vi "SUB SingleTrialPLV_v03.vi"(9 "fc":dbl, 10 "Theta":cluster{"Lat":dbl, "Length":dbl}={"Lat"=5.0, "Length"=60.0}, 11 "Waveform":waveform(dbl)) -> (0 "Instantaneous Phase":waveform(dbl), 1 "phase":dbl[](array[numeric]), 2 "PLV graph":cluster{dbl[], dbl[]}[](graph), 3 "PLV":dbl, 4 "Vector":dbl[](array[numeric]))   [LabVIEW 2017]
panel:
  out "dt":dbl
  in  "N 2":i32
  out "BinSize":i32
  out "N":i32
  out "M":i32
  out "N":i32
  out "y":dbl
  out "x":dbl
  out "PLV graph 2":cluster{dbl[], dbl[]}(graph)
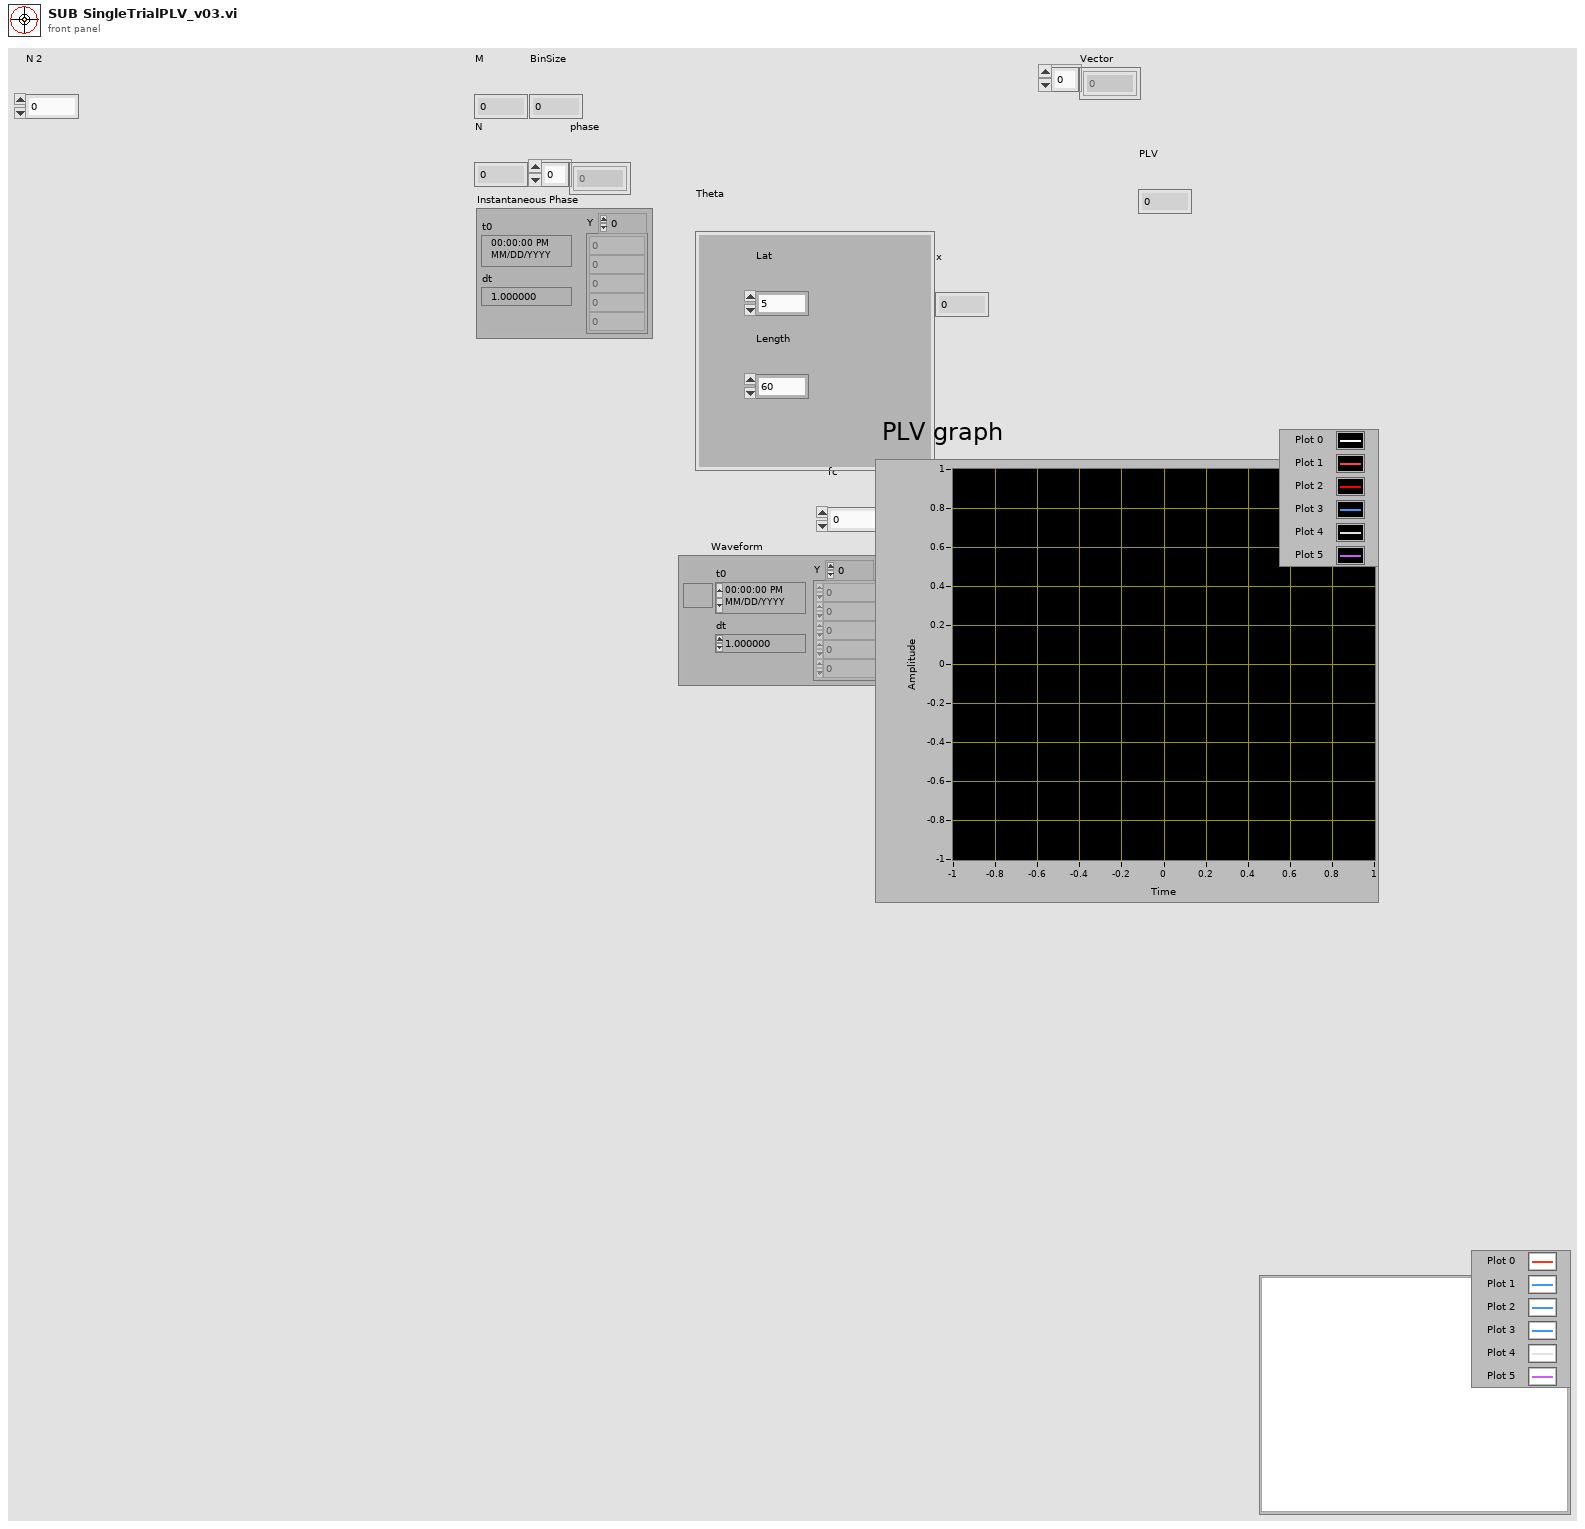
[diagram p1: front panel]
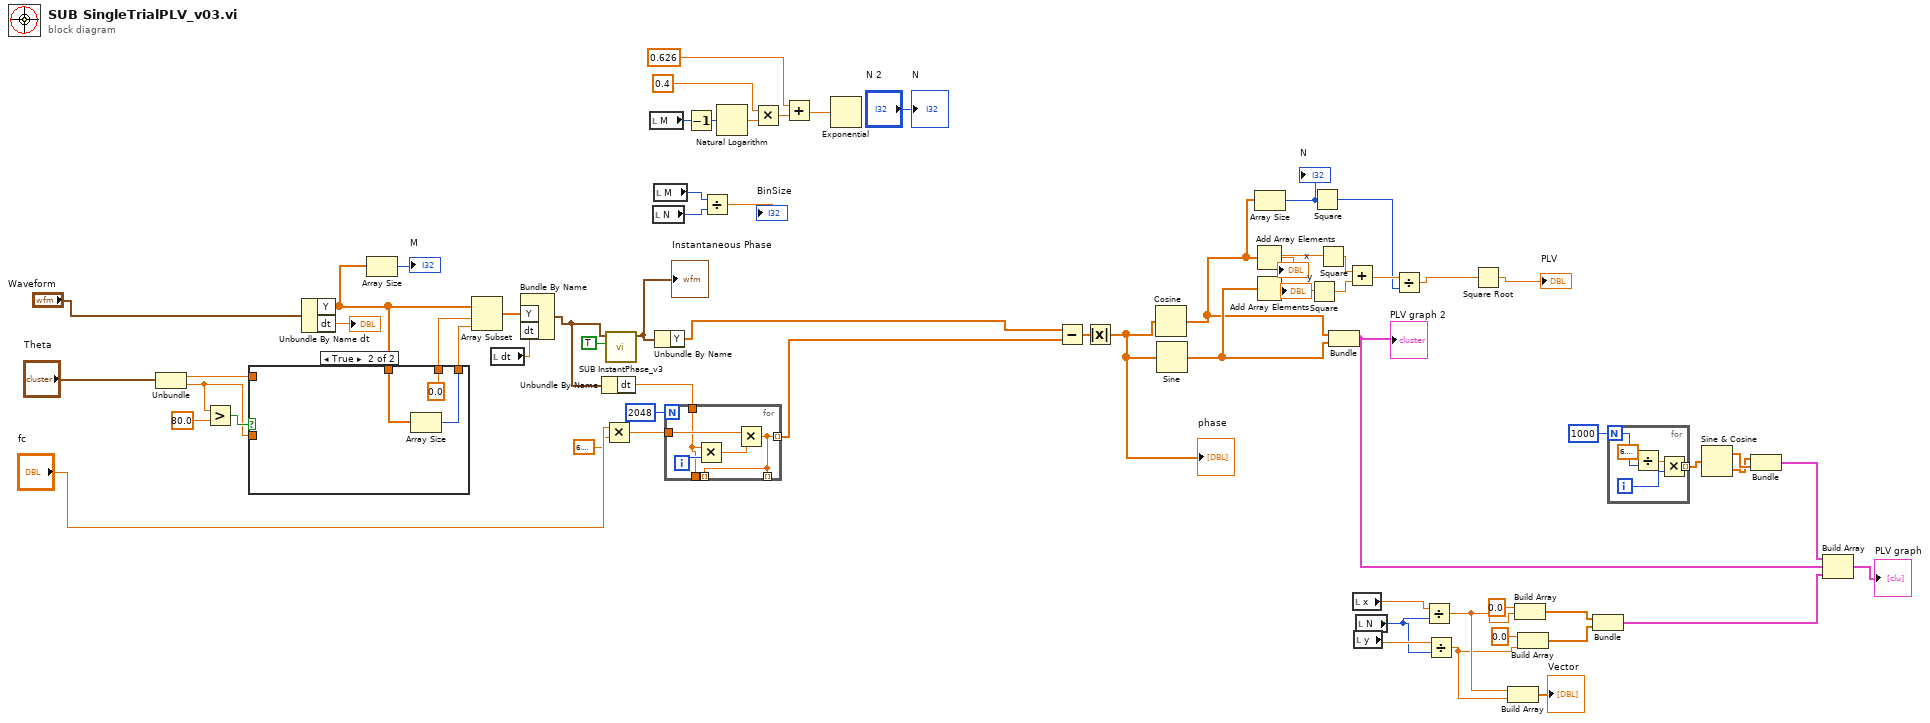
[diagram p0: block diagram]
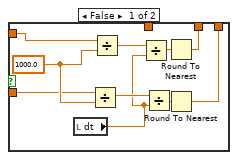
[diagram p2: hidden frame]
diagram:
  n1 = Unbundle("Theta") -> ("Lat"=w47:dbl, "Length"=w6:dbl)
  n2 = Greater?(x=w6, y=80.0) -> (0:w8:bool)
  n3 = Unbundle By Name("Waveform") -> ("Y"=w7:dbl[], "dt"=→"dt":dbl)
  n4 = case shown="True" w8 {
    tunnel: w47 -> [w75 _]
    tunnel: [w69 0.0] -> w46
    tunnel: [w68 w77] -> w43
    tunnel: w7 -> [_ w76]
    tunnel: w6 -> [w66 _]
    frame False {
      w74 = 1000.0 ("y")
      n5 = local read "dt"() -> (w67:dbl)
      n6 = Divide(x=w66, y=w74) -> (x/y=w72:dbl)
      n7 = Divide(x=w75, y=w74) -> (x/y=w73:dbl)
      n8 = Divide(x=w73, y=w67) -> (x/y=w71:dbl)
      n9 = Divide(x=w72, y=w67) -> (x/y=w70:dbl)
      n10 = Round To Nearest(number=w71) -> (nearest integer value=w69:dbl)
      n11 = Round To Nearest(number=w70) -> (nearest integer value=w68:dbl)
    }
    frame True {
      n12 = Array Size(array=w76) -> (size(s)=w77:i32)
    }
  }
  n13 = Array Size(array=w7) -> (size(s)=→"M":i32)
  n14 = Array Subset(array=w7, index=w46, length=w43) -> (w45:dbl[])
  n15 = local read "dt"() -> (w9:dbl)
  n16 = Bundle By Name("Y"=w45, "dt"=w9) -> (w44:waveform(dbl))  [unwired: 1 in]
  n17 = Unbundle By Name(w44) -> ("dt"=w60:dbl)
  n18 = Multiply(x="fc", y=6.283185307179586) -> (x*y=w62:dbl)
  n19 = call "SUB InstantPhase_v3.vi"("Unwrap"=TRUE, "Waveform"=w44) -> ("Instantaneous Phase"=w59:waveform(dbl))  [unwired: 9 in]
  "Instantaneous Phase" <- w59
  n20 = local read "M"() -> (w24:i32)
  n21 = local read "N"() -> (w16:i32)
  n22 = local read "M"() -> (w17:i32)
  n23 = Unbundle By Name(w59) -> ("Y"=w12:dbl[])
  n24 = for {
    N: 2048 -> [_]
    tunnel: w62 -> [w82]
    tunnel: w60 -> [w79]
    tunnel: [w80] -> w13 mode=indexing
    tunnel: [w80] -> _ mode=indexing
    tunnel: [w80] -> _ mode=indexing
    tunnel: [w79] -> _
    i -> [w83]
    n25 = Multiply(x=w79, y=w83) -> (x*y=w81:dbl)
    n26 = Multiply(x=w82, y=w81) -> (x*y=w80:dbl)
  }
  n27 = Decrement(x=w24) -> (x-1=w23:i32)
  n28 = Divide(x=w17, y=w16) -> (x/y=→"BinSize":dbl)
  n29 = Natural Logarithm(1:w23) -> (0:w22:dbl)
  n30 = Multiply(x=0.4, y=w22) -> (x*y=w20:dbl)
  n31 = Add(x=0.626, y=w20) -> (x+y=w18:dbl)
  n32 = Exponential(1:w18) -> ()  [unwired: 1 out]
  n33 = Subtract(x=w12, y=w13) -> (x-y=w58:dbl[])
  n34 = Absolute Value(x=w58) -> (abs(x)=w2:dbl[])
  "phase" <- w2
  n35 = Cosine(x=w2) -> (cos(x)=w51:dbl[])
  n36 = Sine(x=w2) -> (sin(x)=w57:dbl[])
  n37 = Add Array Elements(numeric array=w51) -> (sum=w56:dbl)
  "x" <- w56
  n38 = Add Array Elements(numeric array=w57) -> (sum=w55:dbl)
  "y" <- w55
  n39 = Array Size(array=w51) -> (size(s)=w49:i32)
  "N" <- w49
  n40 = Square(x=w55) -> (x^2=w53:dbl)
  n41 = Square(x=w49) -> (x^2=w48:i32)
  n42 = Square(x=w56) -> (x^2=w54:dbl)
  n43 = Bundle(w51, w57) -> (w35:cluster{dbl[], dbl[]})  [unwired: 1 in]
  "PLV graph 2" <- w35
  n44 = Add(x=w54, y=w53) -> (x+y=w52:dbl)
  n45 = local read "x"() -> (w34:dbl)
  n46 = local read "y"() -> (w28:dbl)
  n47 = local read "N"() -> (w27:i32)
  n48 = Divide(x=w52, y=w48) -> (x/y=w50:dbl)
  n49 = Divide(x=w34, y=w27) -> (x/y=w5:dbl)
  n50 = Divide(x=w28, y=w27) -> (x/y=w4:dbl)
  n51 = Square Root(x=w50) -> (sqrt(x)=→"PLV":dbl)
  n52 = Build Array(w5, w4) -> (→"Vector":dbl[])
  n53 = Build Array(0.0 ("element"), w5) -> (w31:dbl[])
  n54 = Build Array(0.0 ("element"), w4) -> (w30:dbl[])
  n55 = Bundle(w31, w30) -> (w29:cluster{dbl[], dbl[]})  [unwired: 1 in]
  n56 = for {
    N: 1000 -> [w87]
    tunnel: [w86] -> w36 mode=indexing
    i -> [w84]
    n57 = Divide(x=6.283185307179586, y=w87) -> (x/y=w85:dbl)
    n58 = Multiply(x=w85, y=w84) -> (x*y=w86:dbl)
  }
  n59 = Sine & Cosine(0:w36) -> (1:w40:dbl[], 2:w39:dbl[])
  n60 = Bundle(w39, w40) -> (w38:cluster{dbl[], dbl[]})  [unwired: 1 in]
  n61 = Build Array(w38, w35, w29) -> (→"PLV graph":cluster{dbl[], dbl[]}[])
  "N" <- "N 2"
